vi "Start.vi"(8 "error in (no error)":errorcluster, 11 "IThermometer in":refnum<class "IThermometer.lvclass">) -> (0 "error out":errorcluster, 3 "IThermometer out":refnum<class "IThermometer.lvclass">)   [LabVIEW 2023, in "HAL Interfaces.lvlib" / "IThermometer.lvclass"]
uses:
  IThermometer.lvclass
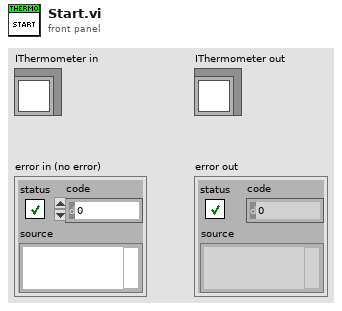
[diagram p1: front panel]
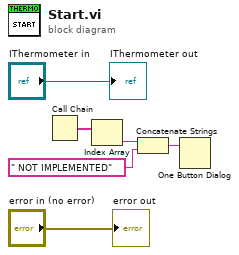
[diagram p0: block diagram]
diagram:
  n1 = Call Chain() -> (call chain=w4:string[])
  n2 = Index Array(array=w4) -> (element=w2:string)  [unwired: 1 in]
  n3 = Concatenate Strings(w2, " NOT IMPLEMENTED" ("string")) -> (w3:string)
  n4 = One Button Dialog(message=w3) -> ()  [unwired: 1 in, 1 out]
  "error out" <- "error in (no error)"
  "IThermometer out" <- "IThermometer in"
